vi "getversion.vi"(11 "Chain IN":bool) -> (1 "Revision":string, 2 "Version":string, 3 "Chain OUT":bool)   [LabVIEW 2010, in "LASA Beta.lvrbt"]
uses:
  LASA Beta.lvrbt
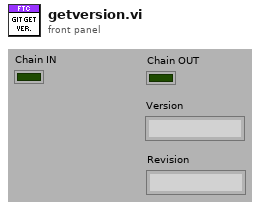
[diagram p1: front panel]
types:
  T1 = typedef "NXT_FileStatusCodes.ctl" = u16
  T2 = typedef "SequenceBoolean.ctl" = bool
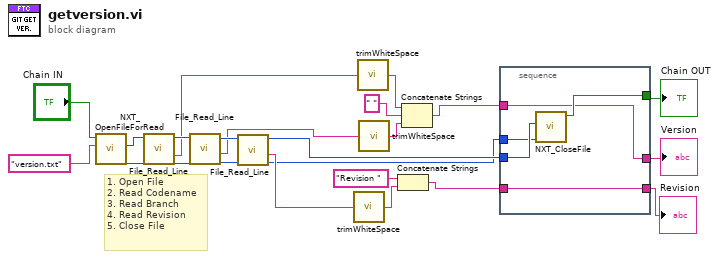
[diagram p0: block diagram]
diagram:
  # "1. Open File\n2. Read Codename\n3. Read Branch\n4. Read Revision\n5. Close File"
  n1 = call <vilib>:"NXT_OpenFileForRead.vi"("Filename"="version.txt", "Sequence Flow in"="Chain IN") -> ("Error out"=w21:T1, "File Handle"=w20:u8)  [unwired: 1 in, 7 out]
  n2 = call <vilib>:"File_Read_Line.vi"("Error In"=w21, "File Handle"=w20) -> ("Error Out"=w17:T1, "Text"=w13:string, "File Handle Out"=w14:u8)  [unwired: 7 out]
  n3 = call <vilib>:"File_Read_Line.vi"("Error In"=w17, "File Handle"=w14) -> ("Error Out"=w9:T1, "Text"=w8:string, "File Handle Out"=w10:u8)  [unwired: 7 out]
  n4 = call <vilib>:"File_Read_Line.vi"("Error In"=w9, "File Handle"=w10) -> ("Error Out"=w1:T1, "Text"=w6:string, "File Handle Out"=w2:u8)  [unwired: 7 out]
  n5 = call <vilib>:"trimWhiteSpace.vi"("string"=w6) -> ("trimmed string"=w5:string)  [unwired: 1 in]
  n6 = call <vilib>:"trimWhiteSpace.vi"("string"=w13) -> ("trimmed string"=w23:string)  [unwired: 1 in]
  n7 = call <vilib>:"trimWhiteSpace.vi"("string"=w8) -> ("trimmed string"=w16:string)  [unwired: 1 in]
  n8 = Concatenate Strings("Revision " ("string"), w5) -> (w4:string)
  n9 = Concatenate Strings(w23, " " ("string"), w16) -> (w11:string)
  n10 = stacked-sequence {
    tunnel: [w28] -> w22
    tunnel: [w27] -> w12
    tunnel: w11 -> [w27]
    tunnel: [w26] -> w3
    tunnel: w4 -> [w26]
    tunnel: w2 -> [w25]
    tunnel: w1 -> [w24]
    frame #0 {
      n11 = call <vilib>:"NXT_CloseFile.vi"("Error in"=w24, "File Handle"=w25) -> ("Sequence Flow out"=w28:T2)  [unwired: 9 out]
    }
  }
  "Chain OUT" <- w22
  "Version" <- w12
  "Revision" <- w3
